vi "GoTo.vi"(5 "PID Gains Angle":T1={"proportional gain (Kc)"=5.0, "integral time (Ti, min)"=0.0, "derivative time (Td, min)"=-2.0}, 6 "Reinitialize":bool, 7 "PID Gains XY":T1={"proportional gain (Kc)"=0.005, "integral time (Ti, min)"=0.0, "derivative time (Td, min)"=-0.07}, 8 "output angle":dbl=4.0, 9 "output xy":dbl=2.7, 10 "Target":dbl[](array[numeric]), 11 "Position":dbl[](array[numeric])) -> (0 "errors":dbl[](array[numeric]), 3 "Output\nVelocity":dbl[](array[numeric]) format="%.2f")   [LabVIEW 2018]
uses:
  <vilib>/Analysis/coordinate.llb/Wrap Angle (scalar).vi
  <vilib>/Analysis/coordinate.llb/2D Cartesian Coordinate Rotation (Scalar).vi
  <vilib>/Analysis/NI_AALPro.lvlib
  <vilib>/Analysis/NI_AAL_Angle.lvlib
panel:
  out "output array":cluster{"output high":dbl, "output low":dbl}[](array[cluster])
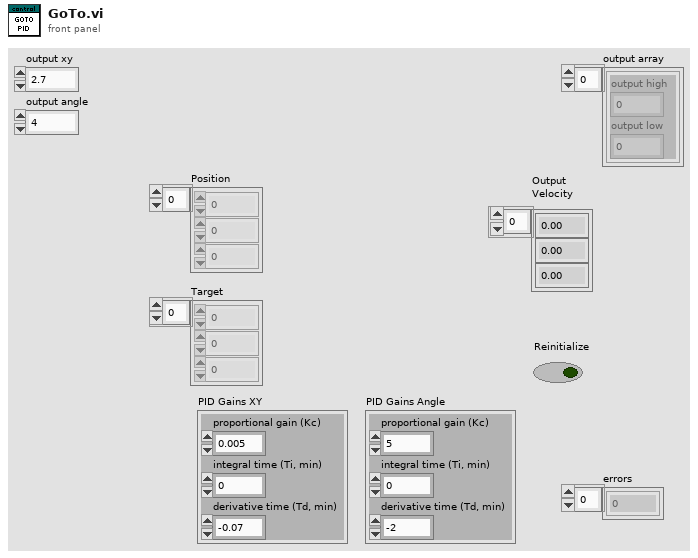
[diagram p1: front panel]
types:
  T1 = cluster{"proportional gain (Kc)":dbl, "integral time (Ti, min)":dbl, "derivative time (Td, min)":dbl}
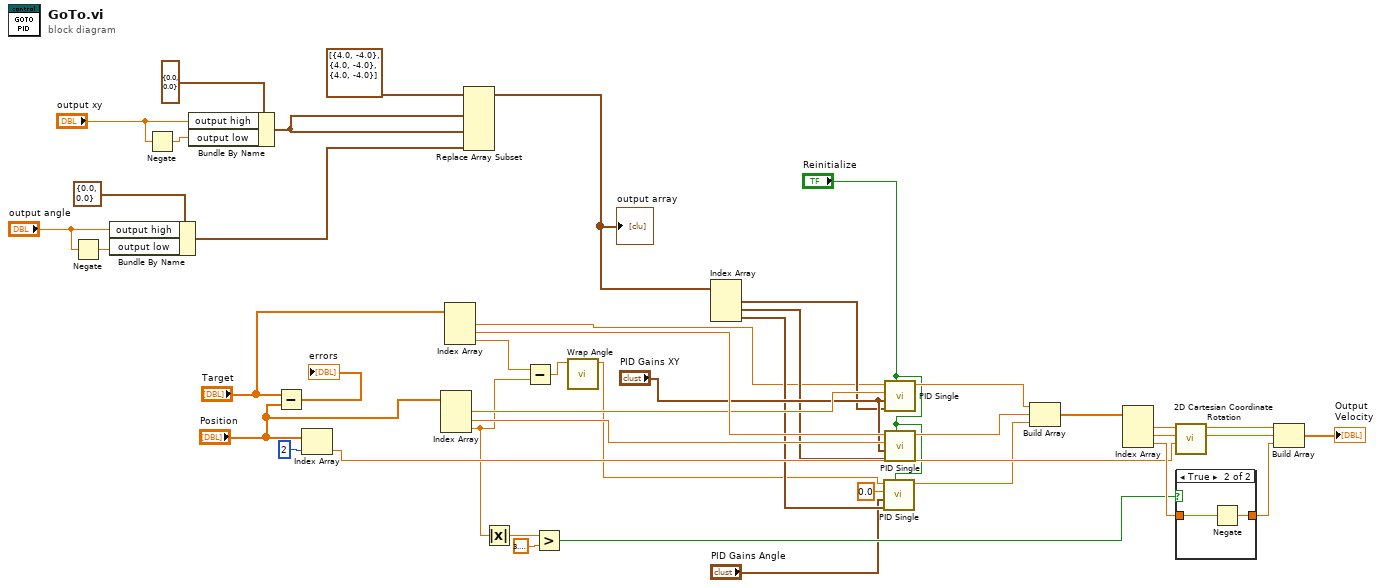
[diagram p0: block diagram]
diagram:
  n1 = Negate(x="output angle") -> (-x=w2:dbl)
  n2 = Bundle By Name(cluster=cluster{"output high":dbl, "output low":dbl} {"output high"=0.0, "output low"=0.0}, "output high"="output angle", "output low"=w2) -> (w8:cluster{"output high":dbl, "output low":dbl})
  n3 = Negate(x="output xy") -> (-x=w4:dbl)
  n4 = Bundle By Name(cluster=cluster{"output high":dbl, "output low":dbl} {"output high"=0.0, "output low"=0.0} ("new element/subarray"), "output high"="output xy", "output low"=w4) -> (w6:cluster{"output high":dbl, "output low":dbl})
  n5 = Subtract(x="Target", y="Position") -> (x-y=→"errors":dbl[])
  n6 = Index Array(array="Position", index=2) -> (element=w35:dbl)
  n7 = Index Array(array="Position") -> (element #1=w25:dbl, element #2=w24:dbl, element #3=w15:dbl)  [unwired: 3 in]
  n8 = Index Array(array="Target") -> (element #1=w17:dbl, element #2=w26:dbl, element #3=w16:dbl)  [unwired: 3 in]
  n9 = Replace Array Subset(array=cluster{"output high":dbl, "output low":dbl}[] [{"output high"=4.0, "output low"=-4.0}, {"output high"=4.0, "output low"=-4.0}, {"output high"=4.0, "output low"=-4.0}] ("output range"), new element #1=w6, new element #2=w6, new element #3=w8) -> (w5:cluster{"output high":dbl, "output low":dbl}[])  [unwired: 3 in]
  "output array" <- w5
  n10 = Absolute Value(x=w15) -> (abs(x)=w39:dbl)
  n11 = Subtract(x=w16, y=w15) -> (x-y=w13:dbl)
  n12 = Greater?(x=w39, y=3.141592653589793) -> (0:w29:bool)
  n13 = call-poly <vilib>:"Wrap Angle.vi"("angle in"=w13) -> ("angle out"=w12:dbl)  [unwired: 9 in, 1 out]
  n14 = Index Array(array=w5) -> (element #1=w21:cluster{"output high":dbl, "output low":dbl}, element #2=w22:cluster{"output high":dbl, "output low":dbl}, element #3=w20:cluster{"output high":dbl, "output low":dbl})  [unwired: 3 in]
  n15 = call "PID Single.vi"("initialize"="Reinitialize", "Limits"=w20, "PID gains in"="PID Gains Angle", "Variable"=0.0, "Setpoint"=w12) -> ("Out"=w31:dbl)  [unwired: 6 in]
  n16 = call "PID Single.vi"("initialize"="Reinitialize", "Limits"=w21, "PID gains in"="PID Gains XY", "Variable"=w25, "Setpoint"=w17) -> ("Out"=w33:dbl)  [unwired: 6 in]
  n17 = call "PID Single.vi"("initialize"="Reinitialize", "Limits"=w22, "PID gains in"="PID Gains XY", "Variable"=w24, "Setpoint"=w26) -> ("Out"=w32:dbl)  [unwired: 6 in]
  n18 = Build Array(w33, w32, w31) -> (w11:dbl[])
  n19 = Index Array(array=w11) -> (element #1=w44:dbl, element #2=w43:dbl, element #3=w38:dbl)  [unwired: 3 in]
  n20 = call-poly <vilib>:"2D Cartesian Coordinate Rotation.vi"("theta"=w35, "y"=w43, "x"=w44) -> ("y out"=w41:dbl, "x out"=w42:dbl)  [unwired: 6 in, 1 out]
  n21 = case shown="True" w29 {
    tunnel: w38 -> [w45 w47]
    tunnel: [w45 w46] -> w37
    frame False {
    }
    frame True {
      n22 = Negate(x=w47) -> (-x=w46:dbl)
    }
  }
  n23 = Build Array(w42, w41, w37) -> (→"Output\nVelocity":dbl[])
